vi "Webcam.vi"(1 "stop":bool) -> (0 "Live Stream":T1(plugin-control))   [LabVIEW 2017]
uses:
  <vilib>/vision/Avi.llb/IMAQ AVI2 Refnum.ctl
  <vilib>/userdefined/High Color/IMAQdx.ctl
  <vilib>/vision/driver/NI_Vision_Acquisition_Software.lvlib
  <resource>/objmgr/imaqdx.rc
panel:
  out "Clock":cluster{dbl, dbl, dbl}(knob)={0.0, 1.701440214160589, 1.7350906402478021} scale=0.012..12.0
  out "# of Pics":dbl
  in  "Snap Picture":bool
  out "path":path
  in  "Record":bool
  out "stop 2":bool
  out "AVI Refnum":T2
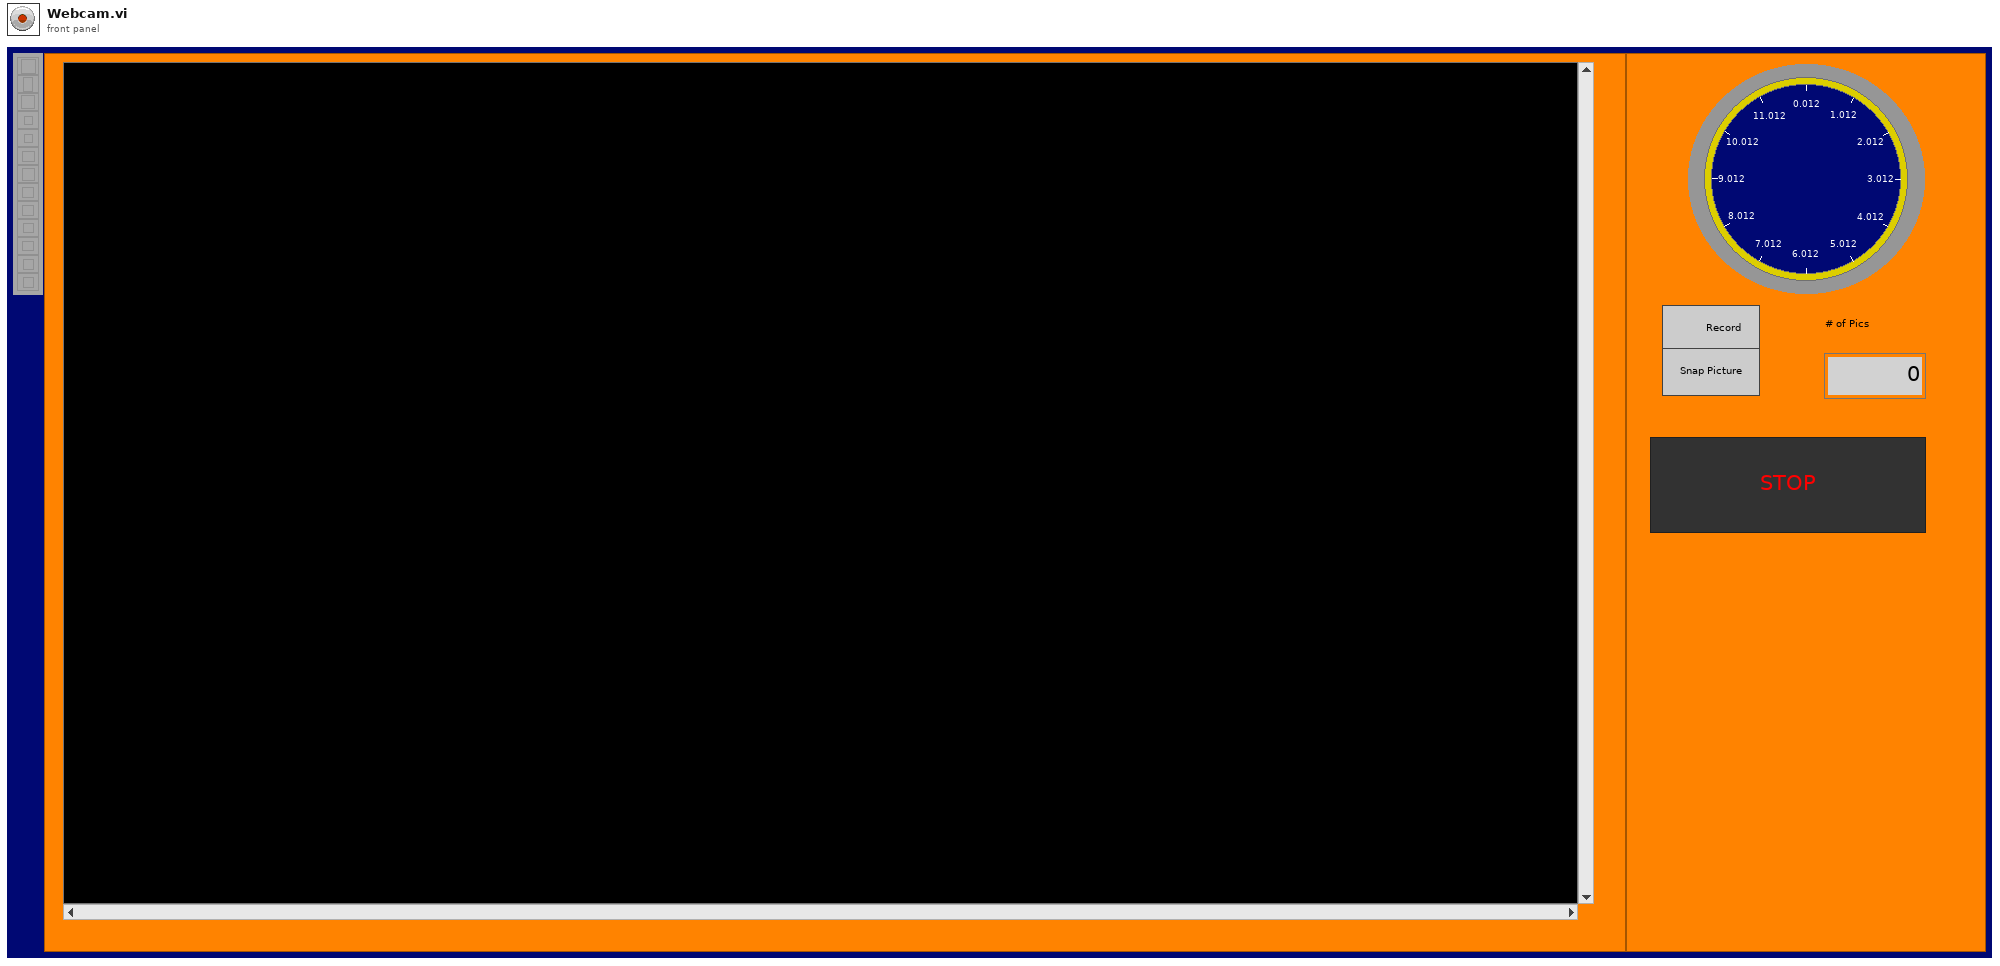
[diagram p1: front panel]
types:
  T1 = typedef "IMAQ Image.ctl" = refnum<image>
  T2 = typedef "IMAQ AVI2 Refnum.ctl" = refnum<k20>
  T3 = typedef "IMAQdx.ctl" = refnum<k21>
  T4 = typedef "Image Type" = u32
  T5 = typedef "LVDateTimeRec.ctl" = cluster{"fractional second":dbl, "second":i32, "minute":i32, "hour":i32, "day of month":i32, "month":i32, "year":i32, "day of week":i32, "day of year":i32, "DST":i32}
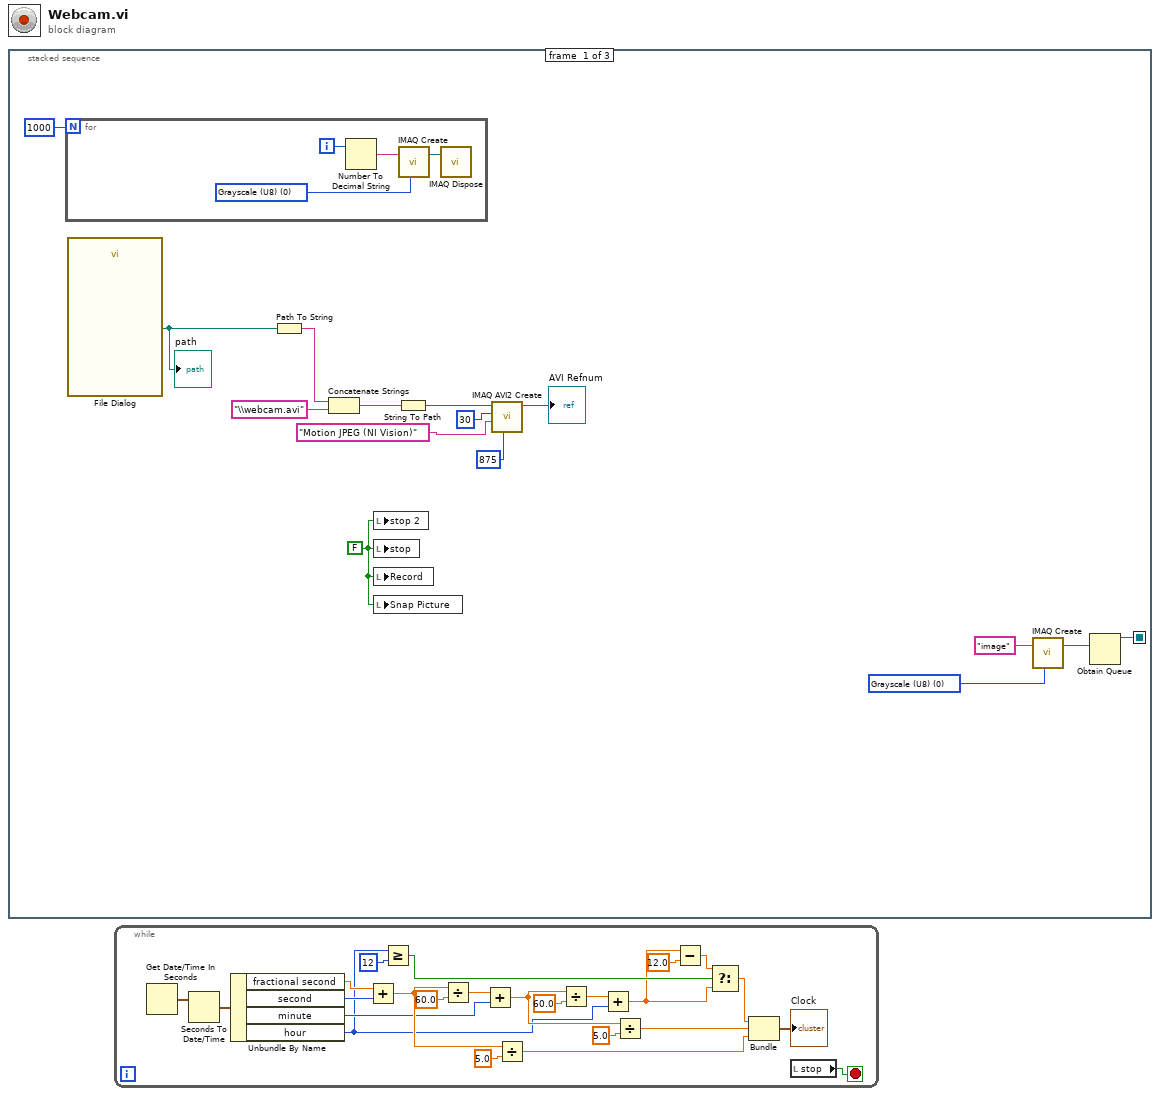
[diagram p0: block diagram]
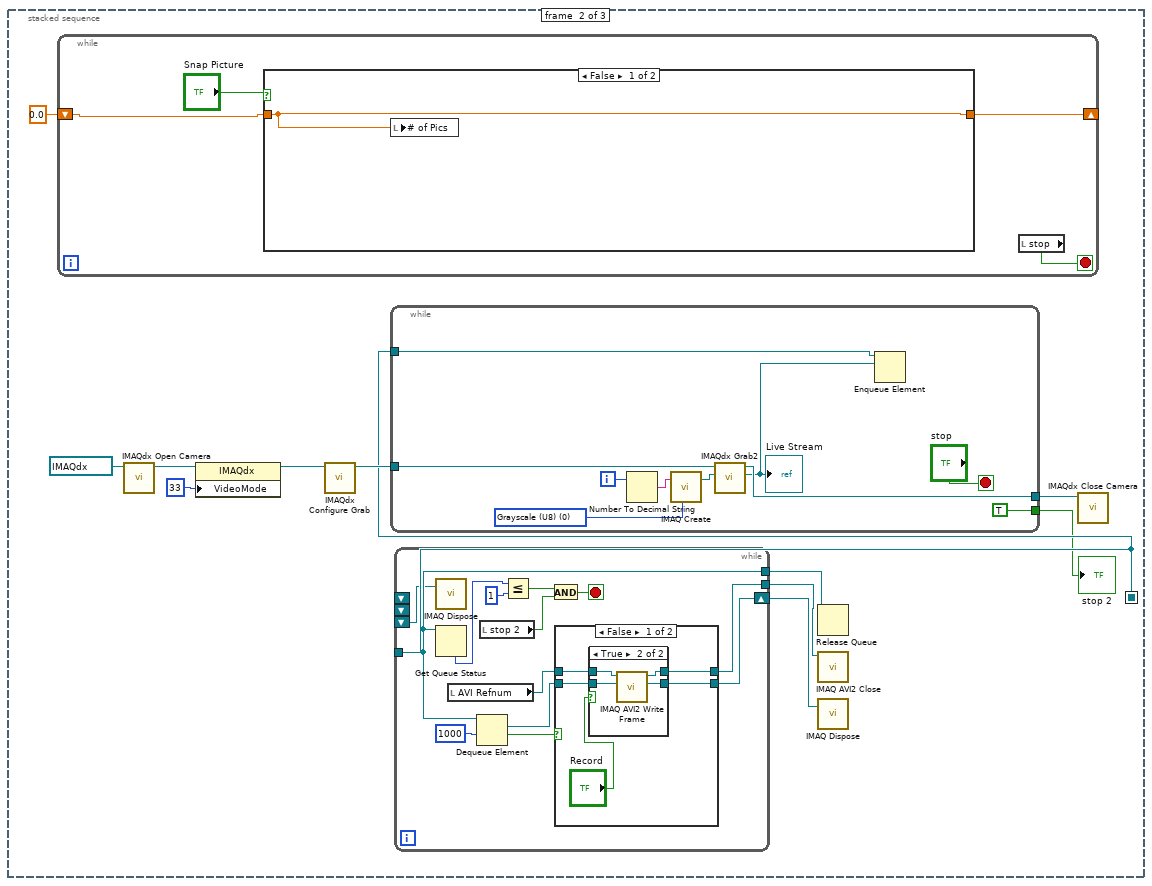
[diagram p2: hidden frame]
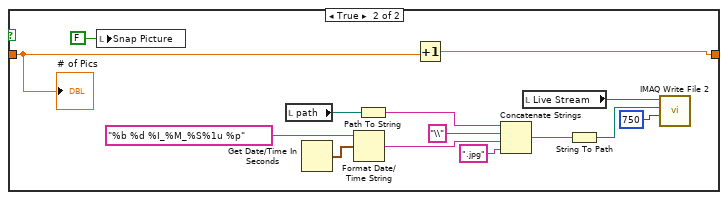
[diagram p3: hidden frame]
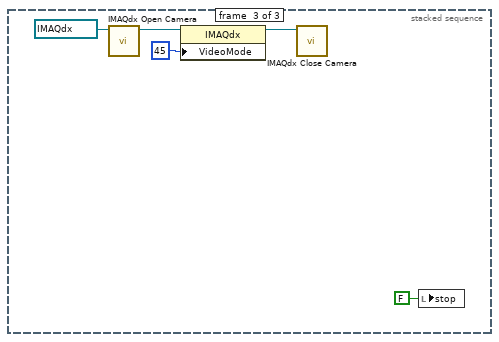
[diagram p6: hidden frame]
diagram:
  n1 = stacked-sequence {
    seq-local: [w8 _ _] -> [_ w27 _]
    frame #0 {
      w2 = FALSE
      w10 = T4 0 items=["Grayscale (U8)", "Grayscale (I16)", "Grayscale (SGL)", "Complex (CSG)", "RGB (U32)", "HSL (U32)", "RGB (U64)", "Grayscale (U16)"] ("Image Type")
      n2 = for {
        N: 1000 -> [_]
        i -> [w19]
        w16 = T4 0 items=["Grayscale (U8)", "Grayscale (I16)", "Grayscale (SGL)", "Complex (CSG)", "RGB (U32)", "HSL (U32)", "RGB (U64)", "Grayscale (U16)"] ("Image Type")
        n3 = Number To Decimal String(number=w19) -> (decimal integer string=w18:string)  [unwired: 1 in]
        n4 = call "IMAQ Create"("Image Name"=w18, "Image Type"=w16) -> ("New Image"=w17:T1)  [unwired: 3 in, 1 out]
        n5 = call "IMAQ Dispose"("Image"=w17) -> ()  [unwired: 5 in, 1 out]
      }
      n6 = call "File Dialog"() -> ("selected path"=w3:path)  [unwired: 12 in, 3 out]
      "path" <- w3
      n7 = Path To String(path=w3) -> (string=w7:string)
      n8 = Concatenate Strings(w7, "\\webcam.avi" ("string")) -> (w5:string)
      n9 = local write "stop 2"(w2) -> ()
      n10 = local write "stop"(w2) -> ()
      n11 = local write "Record"(w2) -> ()
      n12 = local write "Snap Picture"(w2) -> ()
      n13 = String To Path(string=w5) -> (path=w4:path)
      n14 = call "IMAQ AVI2 Create"("Quality"=875, "Codec"="Motion JPEG (NI Vision)", "Frames Per Second"=u32 30, "AVI Path"=w4) -> ("AVI Refnum"=→"AVI Refnum":T2)  [unwired: 6 in, 1 out]
      n15 = call "IMAQ Create"("Image Name"="image", "Image Type"=w10) -> ("New Image"=w11:T1)  [unwired: 3 in, 1 out]
      n16 = Obtain Queue(element data type=w11) -> (queue out=w8:refnum<queue>)  [unwired: 4 in, 2 out]
    }
    frame #1 {
      n17 = while {
        shift-right: [w32] -> _
        shift-left: 0.0 -> [w33]
        stop <- w34 stop-if-true
        n18 = case shown="False" "Snap Picture" {
          tunnel: w33 -> [w36 w39]
          tunnel: [w36 w38] -> w32
          frame False {
            n19 = local write "# of Pics"(w36) -> ()
          }
          frame True {
            n20 = local write "Snap Picture"(FALSE) -> ()
            n21 = local read "path"() -> (w49:path)
            n22 = Get Date/Time In Seconds() -> (seconds since 1Jan1904=w50:timestamp)
            n23 = Format Date/Time String(time format string (%c)="%b %d %I_%M_%S%1u %p", seconds (now)=w50) -> (date/time string=w41:string)  [unwired: 1 in]
            n24 = Path To String(path=w49) -> (string=w43:string)
            n25 = Increment(x=w39) -> (x+1=w38:dbl)
            n26 = Concatenate Strings(w43, "\\" ("string"), w41, ".jpg" ("string")) -> (w40:string)
            n27 = local read "Live Stream"() -> (w44:T1)
            n28 = String To Path(string=w40) -> (path=w45:path)
            n29 = call-poly "IMAQ Write File 2"("Image Quality"=u32 750, "File Path"=w45, "Image"=w44) -> ()  [unwired: 7 in, 2 out]
            "# of Pics" <- w39
          }
        }
        n30 = local read "stop"() -> (w34:bool)
      }
      n31 = call <vilib>:"IMAQdx Open Camera.vi"("Session In"=T3 "cam10") -> ("Session Out"=w20:T3)  [unwired: 9 in, 1 out]
      n32 = property class="IMAQdx"(reference=w20, "VideoMode"=u32 33) -> (reference out=w21:T3)  [unwired: 1 in, 1 out]
      n33 = call <vilib>:"IMAQdx Configure Grab.vi"("Session In"=w21) -> ("Session Out"=w31:T3)  [unwired: 9 in, 1 out]
      n34 = while {
        tunnel: w31 -> [w86]
        tunnel: [w81] -> w28
        tunnel: w27 -> [w79]
        tunnel: [TRUE] -> w24
        i -> [w85]
        stop <- "stop" stop-if-true
        w80 = T4 0 items=["Grayscale (U8)", "Grayscale (I16)", "Grayscale (SGL)", "Complex (CSG)", "RGB (U32)", "HSL (U32)", "RGB (U64)", "Grayscale (U16)"] ("Image Type")
        n35 = Number To Decimal String(number=w85) -> (decimal integer string=w84:string)  [unwired: 1 in]
        n36 = call "IMAQ Create"("Image Name"=w84, "Image Type"=w80) -> ("New Image"=w83:T1)  [unwired: 3 in, 1 out]
        n37 = call <vilib>:"IMAQdx Grab2.vi"("Image In"=w83, "Session In"=w86) -> ("Image Out"=w77:T1, "Session Out"=w81:T3)  [unwired: 6 in, 2 out]
        "Live Stream" <- w77
        n38 = Enqueue Element(queue=w79, element=w77) -> ()  [unwired: 2 in, 3 out]
      }
      "stop 2" <- w24
      n39 = while {
        tunnel: [w60] -> w25
        tunnel: [w56] -> w26
        tunnel: w27 -> [w56]
        shift-right: [w52] -> w23
        shift-left: _ -> [_]
        shift-left: _ -> [_]
        shift-left: _ -> [w51]
        stop <- w57 stop-if-true
        n40 = call "IMAQ Dispose"("Image"=w51) -> ()  [unwired: 5 in, 1 out]
        n41 = Get Queue Status(queue=w56) -> (# elements in queue=w61:i32)  [unwired: 2 in, 7 out]
        n42 = local read "AVI Refnum"() -> (w63:T2)
        n43 = Dequeue Element(queue=w56, timeout in ms (-1)=1000) -> (element=w59:T1, timed out?=w53:bool)  [unwired: 1 in, 2 out]
        n44 = local read "stop 2"() -> (w55:bool)
        n45 = Less Or Equal?(x=w61, y=1) -> (x <= y?=w58:bool)
        n46 = And(x=w58, y=w55) -> (x .and. y?=w57:bool)
        n47 = case shown="False" w53 {
          tunnel: w63 -> [w68 w76]
          tunnel: [w67 w76] -> w60
          tunnel: w59 -> [w66 w75]
          tunnel: [w65 w75] -> w52
          frame False {
            n48 = case shown="True" "Record" {
              tunnel: w68 -> [w69 w74]
              tunnel: [w69 w73] -> w67
              tunnel: w66 -> [w70 w72]
              tunnel: [w70 w71] -> w65
              frame False {
              }
              frame True {
                n49 = call "IMAQ AVI2 Write Frame"("Image"=w72, "AVI Refnum"=w74) -> ("Image Out (duplicate)"=w71:T1, "AVI Refnum (duplicate)"=w73:T2)  [unwired: 7 in, 1 out]
              }
            }
          }
          frame True {
          }
        }
      }
      n50 = Release Queue(queue=w26) -> ()  [unwired: 2 in, 3 out]
      n51 = call "IMAQ AVI2 Close"("AVI Refnum"=w25) -> ()  [unwired: 10 in, 1 out]
      n52 = call "IMAQ Dispose"("Image"=w23) -> ()  [unwired: 5 in, 1 out]
      n53 = call <vilib>:"IMAQdx Close Camera.vi"("Session In"=w28) -> ()  [unwired: 10 in, 1 out]
    }
    frame #2 {
      n54 = call <vilib>:"IMAQdx Open Camera.vi"("Session In"=T3 "cam10") -> ("Session Out"=w90:T3)  [unwired: 9 in, 1 out]
      n55 = property class="IMAQdx"(reference=w90, "VideoMode"=u32 45) -> (reference out=w88:T3)  [unwired: 1 in, 1 out]
      n56 = call <vilib>:"IMAQdx Close Camera.vi"("Session In"=w88) -> ()  [unwired: 10 in, 1 out]
      n57 = local write "stop"(FALSE ("stop")) -> ()
    }
  }
  n58 = while {
    stop <- w115 stop-if-true
    n59 = Get Date/Time In Seconds() -> (seconds since 1Jan1904=w111:timestamp)
    n60 = Seconds To Date/Time(time stamp (now)=w111) -> (date time rec=w112:T5)  [unwired: 1 in]
    n61 = Unbundle By Name(w112) -> ("fractional second"=w113:dbl, "second"=w114:i32, "minute"=w107:i32, "hour"=w98:i32)
    n62 = Add(x=w113, y=w114) -> (x+y=w110:dbl)
    n63 = Greater Or Equal?(x=w98, y=12) -> (x >= y?=w99:bool)
    n64 = Divide(x=w110, y=60.0) -> (x/y=w108:dbl)
    n65 = Add(x=w108, y=w107) -> (x+y=w103:dbl)
    n66 = Divide(x=w110, y=5.0) -> (x/y=w100:dbl)
    n67 = Divide(x=w103, y=60.0) -> (x/y=w101:dbl)
    n68 = Add(x=w101, y=w98) -> (x+y=w95:dbl)
    n69 = Divide(x=w103, y=5.0) -> (x/y=w104:dbl)
    n70 = Subtract(x=w95, y=12.0) -> (x-y=w93:dbl)
    n71 = Select(t=w93, s=w99, f=w95) -> (s? t:f=w96:dbl)
    n72 = Bundle(w96, w104, w100) -> (→"Clock":cluster{dbl, dbl, dbl})  [unwired: 1 in]
    n73 = local read "stop"() -> (w115:bool)
  }
